vi "intro to diy clusters.vi"() -> ()   [LabVIEW 2019]
panel:
  in  "?":bool
  out "output cluster":T1
  in  "Numeric other new value":dbl
  in  "String new value":string
  in  "Numeric new value":dbl
  in  "Boolean new value":bool
  out "String":string
  out "Numeric other 1":dbl
  out "Numeric 1":dbl
  out "Boolean":bool
  in  "Cluster":T1
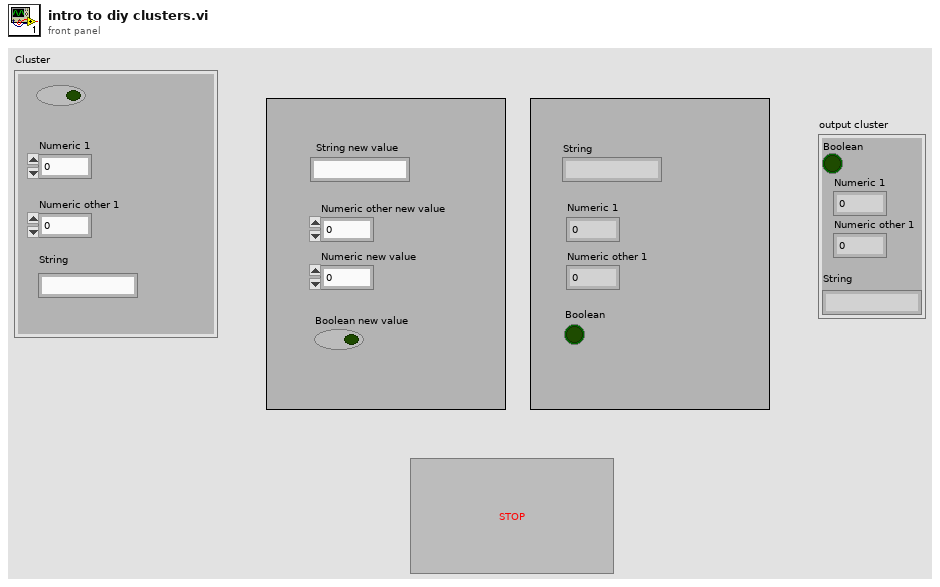
[diagram p1: front panel]
types:
  T1 = cluster{"Boolean":bool, "Numeric 1":dbl, "Numeric other 1":dbl, "\nString":string}
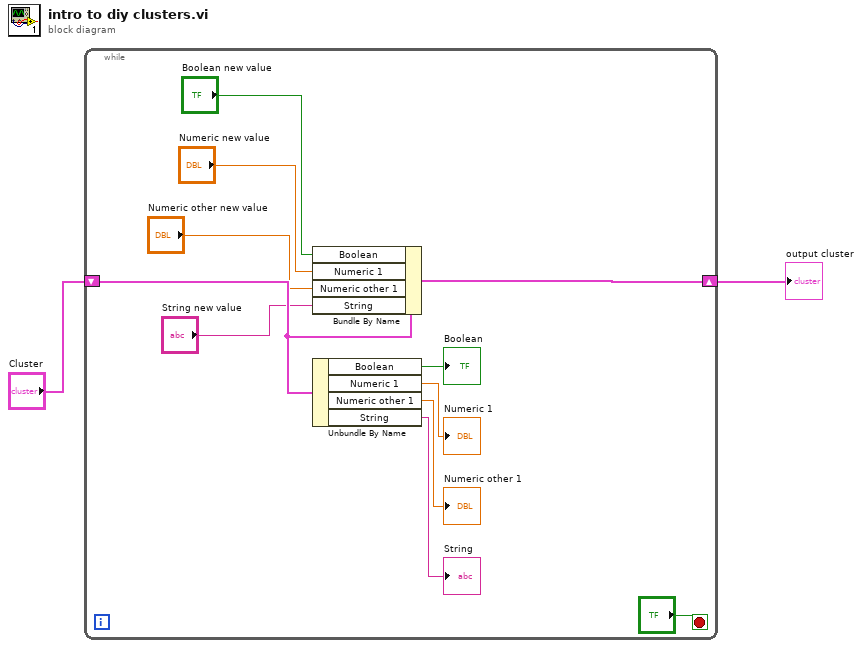
[diagram p0: block diagram]
diagram:
  n1 = while {
    shift-right: [w4] -> w1
    shift-left: "Cluster" -> [w9]
    stop <- "?" stop-if-true
    n2 = Bundle By Name(cluster=w9, "Boolean"="Boolean new value", "Numeric 1"="Numeric new value", "Numeric other 1"="Numeric other new value", "String"="String new value") -> (w4:T1)
    n3 = Unbundle By Name(w9) -> ("Boolean"=→"Boolean":bool, "Numeric 1"=→"Numeric 1":dbl, "Numeric other 1"=→"Numeric other 1":dbl, "String"=→"String":string)
  }
  "output cluster" <- w1
